vi "数据发送test.vi"() -> ()   [LabVIEW 2016, in "数据传输系统.lvlib"]
uses:
  <vilib>/Utility/config.llb/Write Key (String).vi
  <vilib>/Utility/config.llb/NI_LVConfig.lvlib
panel:
  out "数据发送起始时间":timestamp format="%<%.3X\n%Y/%m/%d>T"
  # "根据参数种类来区分"
  # "1.数据\n2.日志\n3.告警\n4.状态"
  # "根据数据时间搜索数据-------判断测量模式------分别进入不同分支"
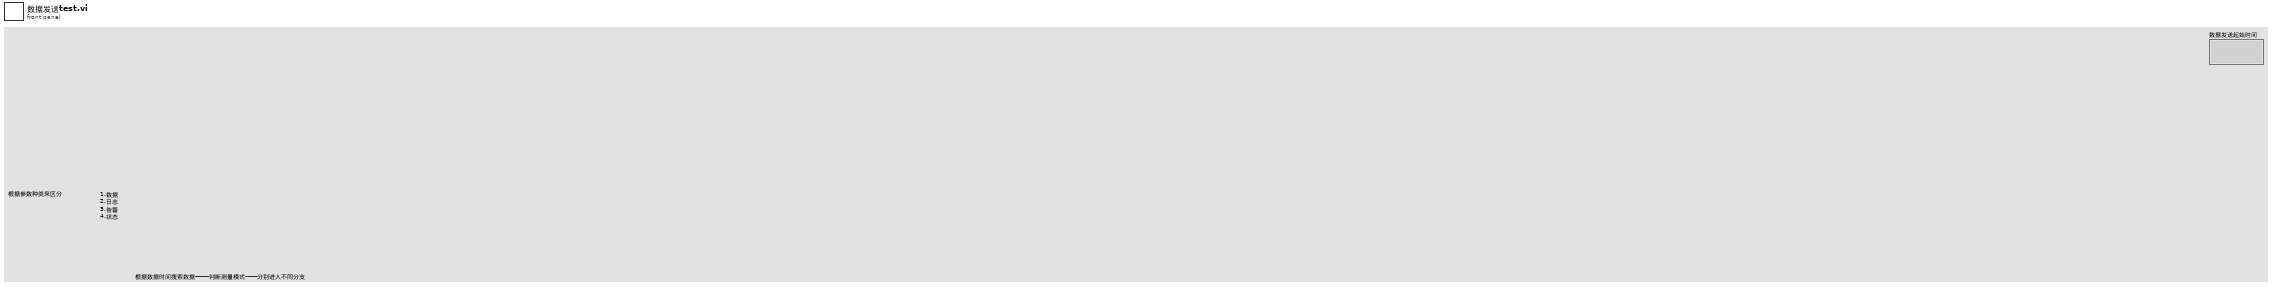
[diagram p1: front panel]
types:
  T1 = cluster{"CODMn":string, "CODCr":string, "DO":string, "铜":string, "PH":string, "氨氮":string, "比电导率":string, "水温":string, "COD":string, "浊度":string, "总氮":string, "总磷":string, "叶绿素a":string, "藻密度":string, "水位":string, "流速":string, "瞬时流量":string, "累积流量":string, "亚硝酸盐":string, "硫化物":string, "ORP":string, "铅":string, "镉":string, "锌":string, "镍":string, "锰":string, "汞":string, "气温":string, "气压":string, "风速":string, "风向":string}
  T2 = cluster{"time1":string, "time2":string, "time3":string, "time4":string, "time5":string, "time6":string, "time7":string, "time8":string, "time9":string, "time10":string, "time11":string, "time12":string, "time13":string, "time14":string, "time15":string, "time16":string, "time17":string, "time18":string, "time19":string, "time20":string, "time21":string, "time22":string, "time23":string, "time24":string, "time25":string, "time26":string, "time27":string, "time28":string, "time29":string, "time30":string, "time31":string}
  T3 = typedef "NI_LVConfig.lvlib/Config Data RefNum.ctl" = refnum<k1>
  T4 = cluster{"水样数据索引[0]":string, "水样数据索引[1]":string, "水样数据索引[2]":string, "水样数据索引[3]":string, "水样数据索引[4]":string, "水样数据索引[5]":string, "水样数据索引[6]":string, "水样数据索引[7]":string, "水样数据索引[8]":string, "水样数据索引[9]":string, "水样数据索引[10]":string, "水样数据索引[11]":string, "水样数据索引[12]":string, "水样数据索引[13]":string, "水样数据索引[14]":string, "水样数据索引[15]":string, "水样数据索引[16]":string, "水样数据索引[17]":string, "水样数据索引[18]":string, "水样数据索引[19]":string, "水样数据索引[20]":string, "水样数据索引[21]":string, "水样数据索引[22]":string, "水样数据索引[23]":string, "水样数据索引[24]":string, "水样数据索引[25]":string, "水样数据索引[26]":string, "水样数据索引[27]":string, "水样数据索引[28]":string, "水样数据索引[29]":string, "水样数据索引[30]":string}
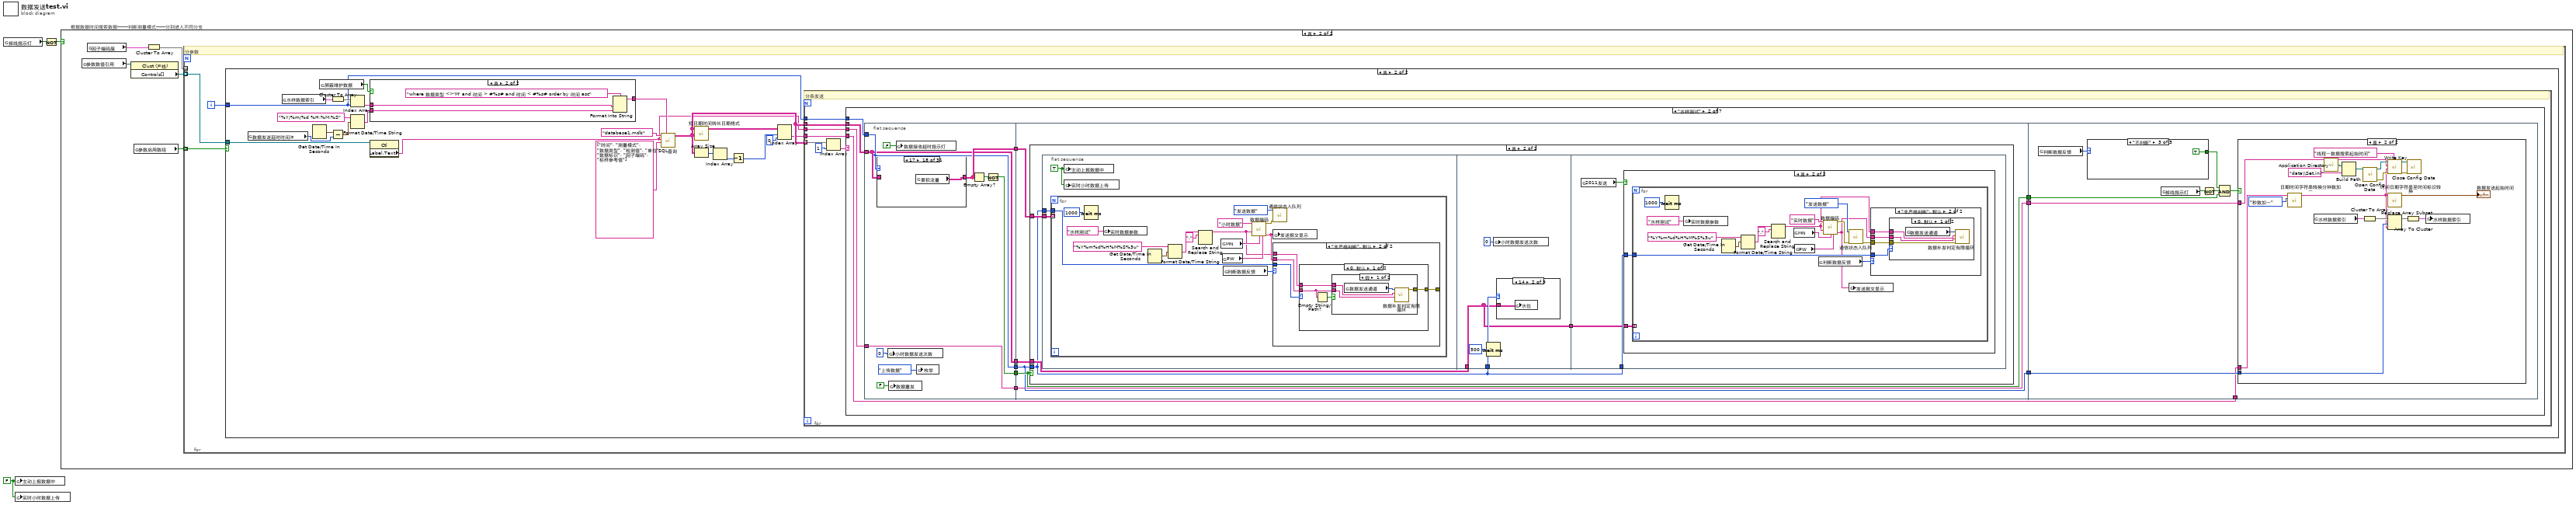
[diagram p0: block diagram]
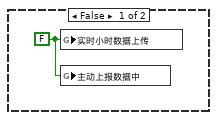
[diagram p2: hidden frame]
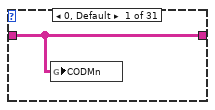
[diagram p5: hidden frame]
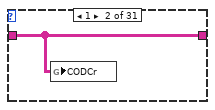
[diagram p6: hidden frame]
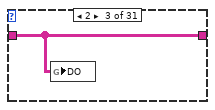
[diagram p7: hidden frame]
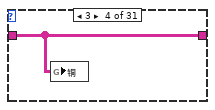
[diagram p8: hidden frame]
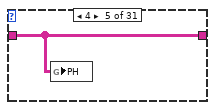
[diagram p9: hidden frame]
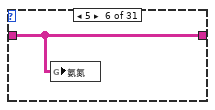
[diagram p10: hidden frame]
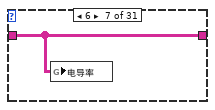
[diagram p11: hidden frame]
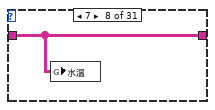
[diagram p12: hidden frame]
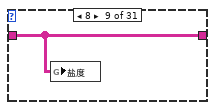
[diagram p13: hidden frame]
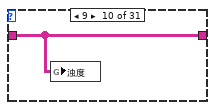
[diagram p14: hidden frame]
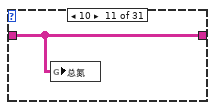
[diagram p15: hidden frame]
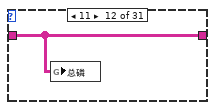
[diagram p16: hidden frame]
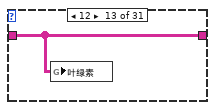
[diagram p17: hidden frame]
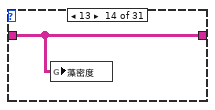
[diagram p18: hidden frame]
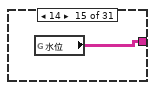
[diagram p19: hidden frame]
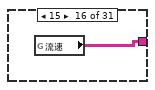
[diagram p20: hidden frame]
diagram:
  w3 = FALSE ("小时数据上传")
  # "根据数据时间搜索数据-------判断测量模式------分别进入不同分支"
  n1 = global read "全局 数据发送重叠.vi" "掉线指示灯"() -> (w2:bool)
  n2 = global write "全局 数据发送重叠.vi" "主动上报数据中"(w3) -> ()
  n3 = global write "全局1.vi" "实时小时数据上传"(w3) -> ()
  n4 = Not(x=w2) -> (.not. x?=w1:bool)
  n5 = case shown="真" w1 {
    frame False {
      w4 = FALSE ("小时数据上传")
      n6 = global write "全局1.vi" "实时小时数据上传"(w4) -> ()
      n7 = global write "全局 数据发送重叠.vi" "主动上报数据中"(w4) -> ()
    }
    frame True {
      n8 = global read "断电保存全局.vi" "参数数值引用"() -> (w8:refnum<vi>)
      n9 = global read "断电保存全局.vi" "因子编码簇"() -> (w9:T1)
      n10 = property class="Clust (严格)"(reference=w8) -> ("Controls[]"=w5:refnum<vi>[])  [unwired: 1 in, 2 out]
      n11 = global read "断电保存全局.vi" "参数启用数组"() -> (w6:bool[])
      n12 = Cluster To Array(cluster=w9) -> (array=w7:string[])
      n13 = for {
        tunnel: w7 -> [_] mode=indexing
        tunnel: w6 -> [w12] mode=indexing
        tunnel: w5 -> [w10] mode=indexing
        i -> [w11]
        # "分参数"
        n14 = case shown="真" w12 {
          tunnel: w11 -> [_ w21]
          tunnel: w10 -> [_ w23]
          frame False {
          }
          frame True {
            n15 = global read "断电保存全局.vi" "数据发送延时时间/s"() -> (w31:i32)
            n16 = global read "全局 水样时间.vi" "水样数据索引"() -> (w33:T2)
            n17 = Get Date/Time In Seconds() -> (seconds since 1Jan1904=w30:timestamp)
            n18 = global read "断电保存全局.vi" "屏蔽维护数据"() -> (w28:bool)
            n19 = Cluster To Array(cluster=w33) -> (array=w34:string[])
            n20 = Subtract(x=w30, y=w31) -> (x-y=w29:timestamp)
            n21 = Index Array(array=w34, index=w21) -> (element=w27:string)
            n22 = Format Date/Time String(time format string (%c)="%Y/%m/%d %H:%M:%S" ("时间格式字符串(%c)"), seconds (now)=w29) -> (date/time string=w26:string)  [unwired: 1 in]
            n23 = case shown="真" w28 {
              tunnel: w27 -> [w207 w212]
              tunnel: w26 -> [w206 w211]
              tunnel: [w208 w210] -> w25
              frame False {
                n24 = Format Into String(format string="where 时间 > #%s# and 时间 < #%s# order by 时间 asc" ("condition"), w207, w206) -> (resulting string=w208:string)  [unwired: 2 in, 1 out]
              }
              frame True {
                n25 = Format Into String(format string="where 数据类型 <>'M' and 时间 > #%s# and 时间 < #%s# order by 时间 asc" ("condition"), w212, w211) -> (resulting string=w210:string)  [unwired: 2 in, 1 out]
              }
            }
            n26 = property class="Ctl"(reference=w23) -> ("Label.Text"=w13:string)  [unwired: 1 in, 2 out]
            n27 = call "SQL查询.vi"("condition"=w25, "columns"=string[] ["时间", "测量模式", "数据类型", "检测值", "单位", "数据标识", "因子编码", "标样参考值"], "table输入"=w13, "database"="database1.mdb") -> ("data"=w15:string[][])  [unwired: 5 in, 2 out]
            n28 = call "短日期时间转长日期格式.vi"("data"=w15) -> ("输出数组"=w20:string[][])  [unwired: 10 in]
            n29 = Array Size(array=w15) -> (size(s)=w19:i32[])
            n30 = Index Array(array=w19) -> (element=w18:i32)  [unwired: 1 in]
            n31 = Decrement(x=w18) -> (x-1=w17:i32)
            n32 = Index Array(array=w20, index (row)=w17, index (col)=0 ("禁用的索引 (列)")) -> (element=w14:string)
            n33 = for {
              tunnel: w15 -> [w41] mode=indexing
              tunnel: w21 -> [w38]
              tunnel: w15 -> [w37]
              tunnel: w14 -> [w36]
              tunnel: w13 -> [w35]
              # "分条发送"
              n34 = Index Array(array=w41, index=1 ("索引")) -> (element=w39:string)
              n35 = case shown="\"水样测试\"" w39 {
                tunnel: w38 -> [_ w53 _ _ _ _ _]
                tunnel: w37 -> [_ w52 _ _ _ _ _]
                tunnel: w36 -> [_ w42 _ _ _ _ _]
                tunnel: w35 -> [_ w45 _ _ _ _ _]
                frame "假", Default {
                }
                frame "水样测试" {
                  n36 = flat-sequence {
                    tunnel: w53 -> [w56]
                    tunnel: w52 -> [w55]
                    tunnel: [w58] -> w51
                    tunnel: [w57] -> w50
                    tunnel: [w56] -> w49
                    tunnel: [w55] -> w48
                    tunnel: w45 -> [w54]
                    tunnel: [w54] -> w43
                    tunnel: w51 -> [w97]
                    tunnel: w50 -> [w99]
                    tunnel: w49 -> [w96]
                    tunnel: w48 -> [w98]
                    tunnel: [w97] -> w47
                    tunnel: [w96] -> w46
                    tunnel: [w95] -> w44
                    tunnel: w43 -> [w95]
                    tunnel: w47 -> [w179]
                    tunnel: w46 -> [w177]
                    tunnel: w44 -> [w176]
                    tunnel: w42 -> [w175]
                    frame #0 {
                      n37 = case shown="17" w56 {
                        tunnel: w55 -> [w64 w65 w66 w67 w68 w69 w70 w71 w72 w73 w74 w75 w76 w77 _ _ _ _ w82 w83 w84 w85 w86 w87 w88 w89 w90 _ _ _ _]
                        tunnel: [w64 w65 w66 w67 w68 w69 w70 w71 w72 w73 w74 w75 w76 w77 w78 w79 w80 w81 w82 w83 w84 w85 w86 w87 w88 w89 w90 w91 w92 w93 w94] -> w57
                        frame 0, Default {
                          n38 = global write "全局 所有参数.vi" "CODMn"(w64) -> ()
                        }
                        frame 1 {
                          n39 = global write "全局 所有参数.vi" "CODCr"(w65) -> ()
                        }
                        frame 2 {
                          n40 = global write "全局 所有参数.vi" "DO"(w66) -> ()
                        }
                        frame 3 {
                          n41 = global write "全局 所有参数.vi" "铜"(w67) -> ()
                        }
                        frame 4 {
                          n42 = global write "全局 所有参数.vi" "PH"(w68) -> ()
                        }
                        frame 5 {
                          n43 = global write "全局 所有参数.vi" "氨氮"(w69) -> ()
                        }
                        frame 6 {
                          n44 = global write "全局 所有参数.vi" "电导率"(w70) -> ()
                        }
                        frame 7 {
                          n45 = global write "全局 所有参数.vi" "水温"(w71) -> ()
                        }
                        frame 8 {
                          n46 = global write "全局 所有参数.vi" "盐度"(w72) -> ()
                        }
                        frame 9 {
                          n47 = global write "全局 所有参数.vi" "浊度"(w73) -> ()
                        }
                        frame 10 {
                          n48 = global write "全局 所有参数.vi" "总氮"(w74) -> ()
                        }
                        frame 11 {
                          n49 = global write "全局 所有参数.vi" "总磷"(w75) -> ()
                        }
                        frame 12 {
                          n50 = global write "全局 所有参数.vi" "叶绿素"(w76) -> ()
                        }
                        frame 13 {
                          n51 = global write "全局 所有参数.vi" "藻密度"(w77) -> ()
                        }
                        frame 14 {
                          n52 = global read "全局 所有参数.vi" "水位"() -> (w78:string[][])
                        }
                        frame 15 {
                          n53 = global read "全局 所有参数.vi" "流速"() -> (w79:string[][])
                        }
                        frame 16 {
                          n54 = global read "全局 所有参数.vi" "瞬时流量"() -> (w80:string[][])
                        }
                        frame 17 {
                          n55 = global read "全局 所有参数.vi" "累积流量"() -> (w81:string[][])
                        }
                        frame 18 {
                          n56 = global write "全局 所有参数.vi" "亚硝酸盐"(w82) -> ()
                        }
                        frame 19 {
                          n57 = global write "全局 所有参数.vi" "硫化物"(w83) -> ()
                        }
                        frame 20 {
                          n58 = global write "全局 所有参数.vi" "ORP"(w84) -> ()
                        }
                        frame 21 {
                          n59 = global write "全局 所有参数.vi" "铅"(w85) -> ()
                        }
                        frame 22 {
                          n60 = global write "全局 所有参数.vi" "镉"(w86) -> ()
                        }
                        frame 23 {
                          n61 = global write "全局 所有参数.vi" "锌"(w87) -> ()
                        }
                        frame 24 {
                          n62 = global write "全局 所有参数.vi" "镍"(w88) -> ()
                        }
                        frame 25 {
                          n63 = global write "全局 所有参数.vi" "锰"(w89) -> ()
                        }
                        frame 26 {
                          n64 = global write "全局 所有参数.vi" "汞"(w90) -> ()
                        }
                        frame 27 {
                          n65 = global read "全局 所有参数.vi" "气温"() -> (w91:string[][])
                        }
                        frame 28 {
                          n66 = global read "全局 所有参数.vi" "气压"() -> (w92:string[][])
                        }
                        frame 29 {
                          n67 = global read "全局 所有参数.vi" "风速"() -> (w93:string[][])
                        }
                        frame 30 {
                          n68 = global read "全局 所有参数.vi" "风向"() -> (w94:string[][])
                        }
                      }
                      n69 = global write "全局 小时数据发送次数.vi" "小时数据发送次数"(0 ("小时数据发送次数")) -> ()
                      n70 = global write "断电保存全局.vi" "数据重发"(FALSE ("数据重发")) -> ()
                      n71 = global write "全局 数据发送重叠.vi" "数据接收超时指示灯"(FALSE ("数据接收超时指示灯")) -> ()
                      n72 = global write "全局1.vi" "枚举"(enum16{"返回请求应答", "上传数据", "返回执行结果"}."上传数据" ("枚举")) -> ()
                      n73 = Empty Array?(array=w57) -> (empty?=w63:bool)
                      n74 = Not(x=w63) -> (.not. x?=w58:bool)
                    }
                    frame #1 {
                      n75 = case shown="真" w97 {
                        tunnel: w99 -> [_ w102]
                        tunnel: w96 -> [_ w100]
                        tunnel: w98 -> [_ w101]
                        frame False {
                        }
                        frame True {
                          n76 = flat-sequence {
                            tunnel: w100 -> [w106]
                            tunnel: w102 -> [w104]
                            tunnel: w100 -> [w136]
                            tunnel: [w134] -> w103
                            tunnel: w101 -> [w134]
                            tunnel: w100 -> [w147]
                            tunnel: w103 -> [w146]
                            frame #0 {
                              w105 = TRUE ("小时数据上传")
                              n77 = for {
                                tunnel: w106 -> [w121]
                                tunnel: w104 -> [_] mode=indexing
                                n78 = Wait (ms)(milliseconds to wait=u32 1000 ("等待时间（毫秒）")) -> ()  [unwired: 1 out]
                                n79 = global write "全局 实时数据参数.vi" "实时数据参数"("水样测试" ("实时数据参数")) -> ()
                                n80 = Get Date/Time In Seconds() -> (seconds since 1Jan1904=w118:timestamp)
                                n81 = Format Date/Time String(time format string (%c)="%Y%m%d%H%M%S%3u" ("时间格式字符串(%c)"), seconds (now)=w118) -> (date/time string=w119:string)  [unwired: 1 in]
                                n82 = Search and Replace String(input string=w119, search string="." ("搜索字符串")) -> (result string=w108:string)  [unwired: 6 in, 3 out]
                                n83 = global read "断电保存全局.vi" "MN"() -> (w114:string)
                                n84 = global read "断电保存全局.vi" "PW"() -> (w113:string)
                                n85 = global read "断电保存全局.vi" "判断数据反馈"() -> (w110:enum16{"非严格判断", "严格判断", "不判断"})
                                n86 = call "数据编码.vi"("table输入"="小时数据" ("新元素/子数组"), "QN"=w108, "MN"=w114, "PW"=w113) -> ("错误常量"=w111:errorcluster, "通讯包字符串"=w109:string)  [unwired: 10 in]
                                n87 = call "通信状态入队列.vi"("错误输入（无错误）"=w111, "枚举"=enum16{"打开连接", "发送数据", "读取数据", "数据处理", "关闭连接"}."发送数据") -> ()  [unwired: 9 in, 1 out]
                                n88 = global write "全局1.vi" "发送报文显示"(w109) -> ()
                                n89 = case shown="\"非严格判断\", 默认" w110 {
                                tunnel: [_ w125] -> _
                                tunnel: w109 -> [_ w124]
                                tunnel: w121 -> [_ w123]
                                tunnel: w108 -> [_ w122]
                                frame "不判断" {
                                }
                                frame "非严格判断", Default {
                                n90 = case shown="0, 默认" w123 {
                                tunnel: [w128 _] -> w125
                                tunnel: w124 -> [w127 _]
                                tunnel: w122 -> [w126 _]
                                frame 0, Default {
                                n91 = Empty String/Path?(string/path=w127) -> (empty?=w129:bool)
                                n92 = case shown="假" w129 {
                                tunnel: [w133 _] -> w128
                                tunnel: w127 -> [w132 _]
                                tunnel: w126 -> [w130 _]
                                frame False {
                                n93 = global read "断电保存全局.vi" "数据发送通道"() -> (w131:enum16{"TCP", "VISA"})
                                n94 = call "数据补发判定有限循环.vi"("数据输入"=w132, "QN"=w130, "数据发送通道"=w131) -> ("error out"=w133:errorcluster)  [unwired: 8 in]
                                }
                                frame True {
                                }
                                }
                                }
                                frame 14..17, 27..30 {
                                }
                                }
                                }
                                }
                              }
                              n95 = global write "全局 数据发送重叠.vi" "主动上报数据中"(w105) -> ()
                              n96 = global write "全局1.vi" "实时小时数据上传"(w105) -> ()
                            }
                            frame #1 {
                              n97 = Wait (ms)(milliseconds to wait=u32 500 ("等待时间（毫秒）")) -> ()  [unwired: 1 out]
                              n98 = global write "全局 小时数据发送次数.vi" "小时数据发送次数"(0 ("小时数据发送次数")) -> ()
                              n99 = case shown="14" w136 {
                                tunnel: w134 -> [_ w138 w139 w140 w141 w142 w143 w144 w145]
                                frame 0, Default {
                                }
                                frame 14 {
                                n100 = global write "全局 所有参数.vi" "水位"(w138) -> ()
                                }
                                frame 15 {
                                n101 = global write "全局 所有参数.vi" "流速"(w139) -> ()
                                }
                                frame 16 {
                                n102 = global write "全局 所有参数.vi" "瞬时流量"(w140) -> ()
                                }
                                frame 17 {
                                n103 = global write "全局 所有参数.vi" "累积流量"(w141) -> ()
                                }
                                frame 27 {
                                n104 = global write "全局 所有参数.vi" "气温"(w142) -> ()
                                }
                                frame 28 {
                                n105 = global write "全局 所有参数.vi" "气压"(w143) -> ()
                                }
                                frame 29 {
                                n106 = global write "全局 所有参数.vi" "风速"(w144) -> ()
                                }
                                frame 30 {
                                n107 = global write "全局 所有参数.vi" "风向"(w145) -> ()
                                }
                              }
                            }
                            frame #2 {
                              n108 = global read "断电保存全局.vi" "2011发送"() -> (w148:bool)
                              n109 = case shown="真" w148 {
                                tunnel: w147 -> [_ w150]
                                tunnel: w146 -> [_ w149]
                                frame False {
                                }
                                frame True {
                                n110 = for {
                                tunnel: w150 -> [w166]
                                tunnel: w149 -> [_] mode=indexing
                                n111 = Wait (ms)(milliseconds to wait=u32 1000 ("等待时间（毫秒）")) -> ()  [unwired: 1 out]
                                n112 = global write "全局 实时数据参数.vi" "实时数据参数"("水样测试" ("实时数据参数")) -> ()
                                n113 = Get Date/Time In Seconds() -> (seconds since 1Jan1904=w154:timestamp)
                                n114 = Format Date/Time String(time format string (%c)="%Y%m%d%H%M%S%3u" ("时间格式字符串(%c)"), seconds (now)=w154) -> (date/time string=w155:string)  [unwired: 1 in]
                                n115 = Search and Replace String(input string=w155, search string="." ("搜索字符串")) -> (result string=w152:string)  [unwired: 6 in, 3 out]
                                n116 = global read "断电保存全局.vi" "MN"() -> (w161:string)
                                n117 = global read "断电保存全局.vi" "PW"() -> (w160:string)
                                n118 = global read "断电保存全局.vi" "判断数据反馈"() -> (w158:enum16{"非严格判断", "严格判断", "不判断"})
                                n119 = call "数据编码.vi"("table输入"="实时数据" ("新元素/子数组"), "QN"=w152, "MN"=w161, "PW"=w160) -> ("错误常量"=w162:errorcluster, "通讯包字符串"=w157:string)  [unwired: 10 in]
                                n120 = call "通信状态入队列.vi"("错误输入（无错误）"=w162, "枚举"=enum16{"打开连接", "发送数据", "读取数据", "数据处理", "关闭连接"}."发送数据") -> ("错误输出"=w159:errorcluster)  [unwired: 9 in]
                                n121 = global write "全局1.vi" "发送报文显示"(w157) -> ()
                                n122 = case shown="\"非严格判断\", 默认" w158 {
                                tunnel: w157 -> [_ w170]
                                tunnel: w159 -> [_ w169]
                                tunnel: w166 -> [_ w168]
                                tunnel: w152 -> [_ w167]
                                frame "不判断" {
                                }
                                frame "非严格判断", Default {
                                n123 = case shown="0, 默认" w168 {
                                tunnel: w170 -> [w174 _]
                                tunnel: w169 -> [w173 _]
                                tunnel: w167 -> [w171 _]
                                frame 0, Default {
                                n124 = global read "断电保存全局.vi" "数据发送通道"() -> (w172:enum16{"TCP", "VISA"})
                                n125 = call "数据补发判定有限循环.vi"("错误输入（无错误）"=w173, "数据输入"=w174, "QN"=w171, "数据发送通道"=w172) -> ()  [unwired: 7 in, 1 out]
                                }
                                frame 14..17, 27..30 {
                                }
                                }
                                }
                                }
                                }
                                }
                              }
                            }
                          }
                        }
                      }
                    }
                    frame #2 {
                      n126 = global read "断电保存全局.vi" "判断数据反馈"() -> (w182:enum16{"非严格判断", "严格判断", "不判断"})
                      n127 = case shown="\"不判断\"" w182 {
                        tunnel: [TRUE w185 TRUE] -> w183
                        frame "非严格判断", Default {
                        }
                        frame "严格判断" {
                          n128 = global read "全局 数据发送重叠.vi" "数据接收超时指示灯"() -> (w186:bool)
                          n129 = Not(x=w186) -> (.not. x?=w185:bool)
                        }
                        frame "不判断" {
                        }
                      }
                      n130 = global read "全局 数据发送重叠.vi" "掉线指示灯"() -> (w181:bool)
                      n131 = Not(x=w181) -> (.not. x?=w178:bool)
                      n132 = Compound Arithmetic op=AND ("复合运算")(w183, w178, w179) -> (w180:bool)
                      n133 = case shown="真" w180 {
                        tunnel: w175 -> [_ w196]
                        tunnel: w177 -> [_ w190]
                        tunnel: w176 -> [_ w197]
                        frame False {
                        }
                        frame True {
                          n134 = call "日期时间字符串转换分钟数加一.vi"("枚举"=enum16{"分钟数加一", "秒数加一", "小时数加一"}."秒数加一", "data[0]"=w196) -> ("日期/时间字符串"=w189:string)  [unwired: 9 in]
                          n135 = global read "全局 水样时间.vi" "水样数据索引"() -> (w191:T2)
                          n136 = call <vilib>:"Application Directory.vi"() -> ("Application Directory"=w198:path)
                          n137 = Build Path(base path=w198, name or relative path="data\\Set.ini" ("名称或相对路径")) -> (appended path=w200:path)
                          n138 = Cluster To Array(cluster=w191) -> (array=w192:string[])
                          n139 = call <vilib>:"Open Config Data.vi"("configuration file path"=w200) -> ("error out"=w202:errorcluster, "refnum"=w201:T3)  [unwired: 8 in, 1 out]
                          n140 = call-poly <vilib>:"Write Key.vi"("section"="线程一数据搜索起始时间", "error in (no error)"=w202, "value"=w189, "key"=w197, "refnum"=w201) -> ("error out"=w204:errorcluster, "refnum out"=w203:T3)  [unwired: 4 in, 1 out]
                          n141 = call "时间日期字符串至时间标识转换.vi"("时间日期字符串"=w189) -> ("时间标识"=→"数据发送起始时间":timestamp)  [unwired: 10 in]
                          n142 = Replace Array Subset(array=w192, new element=w189, index=w190) -> (w193:string[])
                          n143 = Array To Cluster(array=w193) -> (cluster=w194:T4)
                          n144 = call <vilib>:"Close Config Data.vi"("error in (no error)"=w204, "refnum"=w203) -> ()  [unwired: 8 in, 2 out]
                          n145 = global write "全局 水样时间.vi" "水样数据索引"(w194) -> ()
                        }
                      }
                    }
                  }
                }
                frame "空白测试", "零点核查" {
                }
                frame "跨度核查" {
                }
                frame "标样核查" {
                }
                frame "集成干预测试" {
                }
                frame "平行样测试" {
                }
              }
            }
          }
        }
      }
    }
  }
